vi "tcp_getpos.vi"(8 "error in (no error)":errorcluster, 10 "Axis":string(combo), 11 "IP address":string="172.16.6.101") -> (0 "error out":errorcluster, 2 "position":dbl format="%#.10f", 3 "IP address out":string="172.16.6.101")   [LabVIEW 2017]
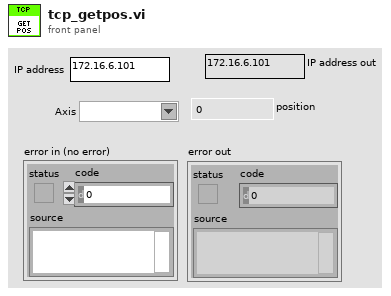
[diagram p1: front panel]
types:
  T1 = cluster{"status":bool, "code":i32, "response":string}
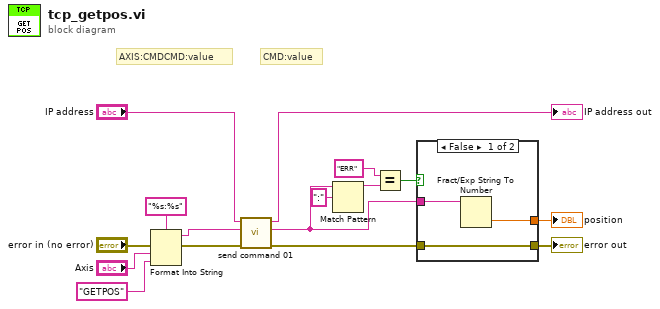
[diagram p0: block diagram]
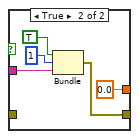
[diagram p2: hidden frame]
diagram:
  # "CMD:value"
  # "AXIS:CMDCMD:value"
  n1 = Format Into String(format string="%s:%s", error in="error in (no error)", "Axis", "GETPOS" ("input 2")) -> (resulting string=w13:string, error out=w12:errorcluster)  [unwired: 1 in]
  n2 = call "send command 01.vi"("error in (no error)"=w12, "command"=w13, "IP address in"="IP address") -> ("error out"=w4:errorcluster, "response"=w1:string, "IP address out"=→"IP address out":string)  [unwired: 6 in]
  n3 = Match Pattern(string=w1, regular expression=":") -> (before substring=w7:string)  [unwired: 1 in, 3 out]
  n4 = Equal?(x="ERR", y=w7) -> (x = y?=w3:bool)
  n5 = case shown="False" w3 {
    tunnel: w1 -> [w18 w22]
    tunnel: [w19 w21] -> w5
    tunnel: w4 -> [w19 _]
    tunnel: [w17 0.0] -> w2
    frame False {
      n6 = Fract/Exp String To Number(string=w18) -> (number=w17:dbl)  [unwired: 3 in, 1 out]
    }
    frame True {
      n7 = Bundle("status"=TRUE, "code"=1, "response"=w22) -> (w21:T1)  [unwired: 1 in]
    }
  }
  "error out" <- w5
  "position" <- w2
